vi "Get all the Controls and Indicators.vi"(0 "Controls[]":refnum<vi>[](array[refnum]), 11 "error in (no error)":errorcluster) -> (4 "Controls[]":refnum<vi>[](array[refnum]), 6 "Indicators[]":refnum<vi>[](array[refnum]), 15 "error out":errorcluster)   [LabVIEW 2021, in "Migrator.lvlib"]
uses:
  Migrator.lvlib
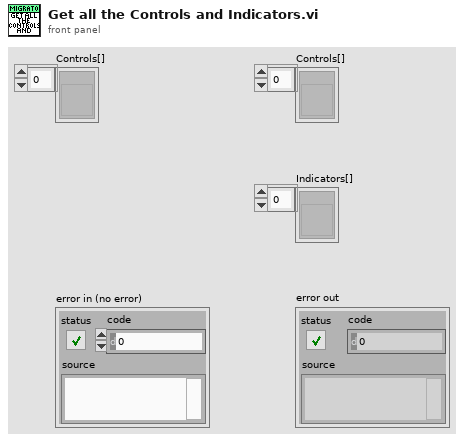
[diagram p1: front panel]
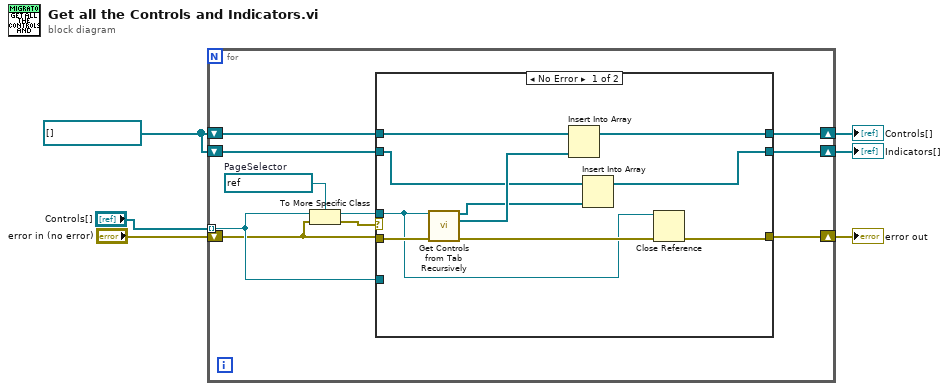
[diagram p0: block diagram]
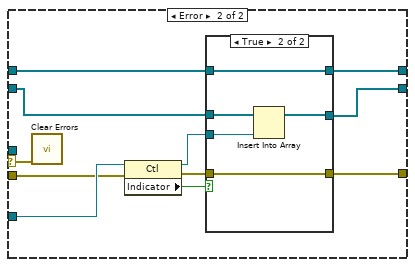
[diagram p2: hidden frame]
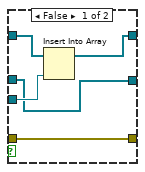
[diagram p3: hidden frame]
diagram:
  w2 = refnum<vi>[] []
  n1 = for {
    tunnel: "Controls[]" -> [w13] mode=indexing
    shift-right: [w9] -> w3
    shift-left: w2 -> [w12]
    shift-right: [w10] -> w4
    shift-left: w2 -> [w11]
    shift-right: [w7] -> w1
    shift-left: "error in (no error)" -> [w8]
    w16 = refnum<vi> refnum  # PageSelector
    n2 = To More Specific Class(target class=w16, reference=w13, error in=w8) -> (specific class reference=w14:refnum<vi>, error out=w15:errorcluster)
    n3 = case shown="No Error" w15 {
      selector: w15 -> [_ w29]
      tunnel: w14 -> [w18 _]
      tunnel: w13 -> [_ w34]
      tunnel: w12 -> [w22 w35]
      tunnel: w11 -> [w25 w36]
      tunnel: [w24 w31] -> w10
      tunnel: [w21 w32] -> w9
      tunnel: w8 -> [w20 w28]
      tunnel: [w17 w27] -> w7
      frame No Error {
        n4 = call "Get Controls from Tab Recursively.vi"("PageSel Refnum"=w18, "error in (no error)"=w20) -> ("Indicators in Tab"=w23:refnum<vi>[], "Controls in Tab"=w26:refnum<vi>[], "error out"=w19:errorcluster)  [unwired: 11 in]
        n5 = Insert Into Array(array=w25, new element=w26) -> (w24:refnum<vi>[])  [unwired: 1 in]
        n6 = Insert Into Array(array=w22, new element=w23) -> (w21:refnum<vi>[])  [unwired: 1 in]
        n7 = Close Reference(reference=w18, error in (no error)=w19) -> (error out=w17:errorcluster)
      }
      frame Error {
        n8 = call <vilib>:"Clear Errors.vi"("error in (no error)"=w29) -> ()  [unwired: 5 in, 2 out]
        n9 = property class="Ctl"(reference=w34, error in=w28) -> (reference out=w33:refnum<vi>, error out=w30:errorcluster, "Indicator"=w37:bool)
        n10 = case shown="True" w37 {
          tunnel: w36 -> [w42 w44]
          tunnel: w35 -> [w39 w47]
          tunnel: w33 -> [w41 w46]
          tunnel: [w39 w45] -> w32
          tunnel: [w40 w44] -> w31
          tunnel: w30 -> [w38 w43]
          tunnel: [w38 w43] -> w27
          frame False {
            n11 = Insert Into Array(array=w42, new element=w41) -> (w40:refnum<vi>[])  [unwired: 1 in]
          }
          frame True {
            n12 = Insert Into Array(array=w47, new element=w46) -> (w45:refnum<vi>[])  [unwired: 1 in]
          }
        }
      }
    }
  }
  "Controls[]" <- w4
  "Indicators[]" <- w3
  "error out" <- w1
